vi "Read Enable Server Generic UE.vi"(11 "Template Server in":refnum<class "Simple_server.lvclass">) -> (2 "Enable Server Generic UE":bool, 3 "Template Server out":refnum<class "Simple_server.lvclass">)   [LabVIEW 2019, in "Simple_server.lvlib" / "Simple_server.lvclass"]
uses:
  Simple_server.lvclass
  Simple_server.lvclass/Simple_server.ctl
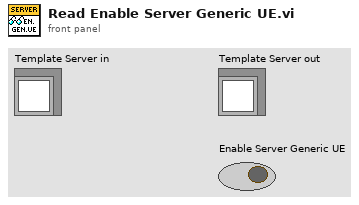
[diagram p1: front panel]
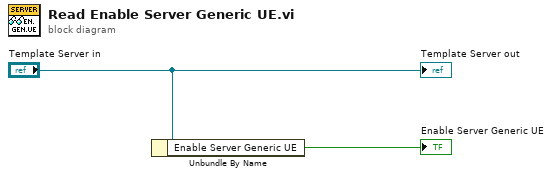
[diagram p0: block diagram]
diagram:
  n1 = Unbundle By Name("Template Server in") -> ("Enable Server Generic UE"=→"Enable Server Generic UE":bool)
  "Template Server out" <- "Template Server in"
